vi "Helmholtz2D_Cal RHS_F Edge.vi"(10 "Domain":T1={"x"={"start x"=0.0, "end x"=1.0, "# of x-points"=11}, "y"={"start y"=0.0, "end y"=1.0, "# of y-points"=11}}, 11 "F(x, y)":dbl[][](array[numeric])) -> (0 "F End Y":dbl[](array[numeric]), 1 "F Start Y":dbl[](array[numeric]), 2 "F End X":dbl[](array[numeric]), 3 "F Start X":dbl[](array[numeric]))   [LabVIEW 2020, in "NI_PDE.lvlib"]
uses:
  <vilib>/gmath/NI_PDE.lvlib
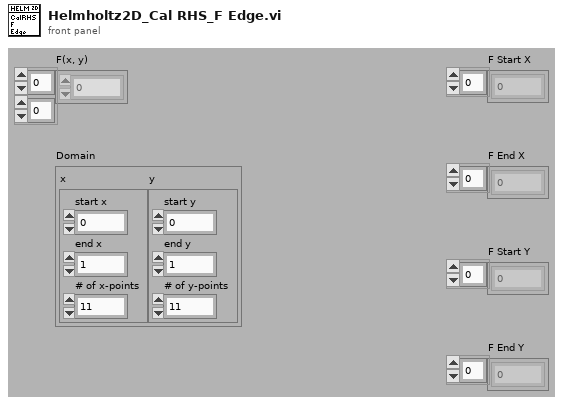
[diagram p1: front panel]
types:
  T1 = cluster{"x":cluster{"start x":dbl, "end x":dbl, "# of x-points":i32}, "y":cluster{"start y":dbl, "end y":dbl, "# of y-points":i32}}
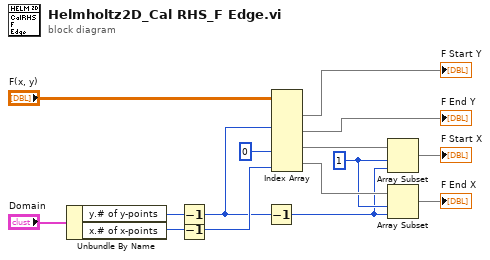
[diagram p0: block diagram]
diagram:
  w5 = 1 ("index")
  n1 = Unbundle By Name("Domain") -> ("y.# of y-points"=w13:i32, "x.# of x-points"=w11:i32)
  n2 = Decrement(x=w13) -> (x-1=w1:i32)
  n3 = Decrement(x=w11) -> (x-1=w3:i32)
  n4 = Decrement(x=w1) -> (x-1=w2:i32)
  n5 = Index Array(array="F(x, y)", index (row) #2=w1, index (col) #3=0 ("disabled index (col)"), index (col) #4=w3) -> (element #1=→"F Start Y":dbl[], element #2=→"F End Y":dbl[], element #3=w8:dbl[], element #4=w6:dbl[])  [unwired: 5 in]
  n6 = Array Subset(array=w8, index=w5, length=w2) -> (→"F Start X":dbl[])
  n7 = Array Subset(array=w6, index=w5, length=w2) -> (→"F End X":dbl[])
